vi "remote.Abort Session.vi"(8 "error in (no error)":errorcluster, 11 "SLSC Remote in":refnum<class "SLSC Interface.lvclass">) -> (0 "error out":errorcluster, 3 "SLSC Remote out":refnum<class "SLSC Interface.lvclass">)   [LabVIEW 2016, in "SLSC Interface.lvclass"]
uses:
  SLSC Interface Class/SLSC Interface.lvclass
  SLSC Interface Class/SLSC Interface.lvclass/SLSC Interface.ctl
  SLSC Interface Class/Read client handle.vi
  SLSC Interface Class/Read URL.vi
  <vilib>/NI/JSON Support for LabVIEW/JSON Data Classes/JSON Object/JSON Object.lvclass
  C:/Program Files (x86)/National Instruments/LabVIEW 2016/vi.lib/NI/JSON Support for LabVIEW/JSON Data Classes/JSON Datatype/JSON Null.lvclass
  SLSC Interface Class/Read session.vi
  <vilib>/NI/JSON Support for LabVIEW/JSON Data Classes/JSON Object/New JSON Object (Empty).vi
  <vilib>/NI/JSON Support for LabVIEW/JSON Data Classes/JSON Object/Insert Key Value Pair (Single String).vi
  <vilib>/NI/NI JSONRPC Server Framework/Classes/Server/Format Client Request (Auto-Increment).vi
  <vilib>/httpClient/POSTBuffer.vi
  <vilib>/NI/NI JSONRPC Server Framework/Classes/Server/Parse Response (Object).vi
  <vilib>/NI/NI JSONRPC Server Framework/Classes/Server/JSONRPC Server.lvclass
  <vilib>/httpClient/LabVIEWHTTPClient.lvlib
  <vilib>/NI/JSON Support for LabVIEW/JSON Data Classes/JSON Helper/JSON Helper.lvclass
  C:/Program Files (x86)/National Instruments/LabVIEW 2016/vi.lib/NI/JSON Support for LabVIEW/JSON Data Classes/JSON Structured Type/JSON Structure.lvclass
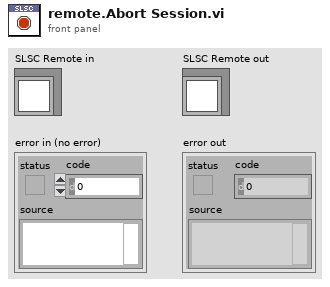
[diagram p1: front panel]
types:
  T1 = typedef "LabVIEWHTTPClient.lvlib/ClientHandle.ctl" = refnum<k1>
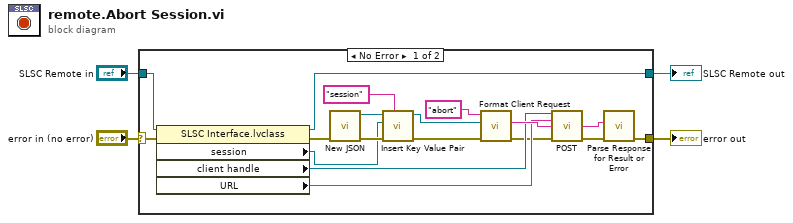
[diagram p0: block diagram]
diagram:
  n1 = case shown="No Error" "error in (no error)" {
    selector: "error in (no error)" -> [w20 w23]
    tunnel: "SLSC Remote in" -> [w22 w24]
    tunnel: [w21 w24] -> w2
    tunnel: [w8 w23] -> w1
    frame No Error {
      n2 = property class="SLSC Interface.lvclass"(reference=w22, error in=w20) -> (reference out=w21:refnum<class "SLSC Interface.lvclass">, error out=w19:errorcluster, "session"=w7:refnum<k21>, "client handle"=w13:T1, "URL"=w12:string)
      n3 = call-poly <vilib>:"New JSON.vi"("error in (no error)"=w19) -> ("error out"=w18:errorcluster, "JSON Object out"=w5:refnum<class "JSON Object.lvclass">)  [unwired: 9 in]
      n4 = call-poly <vilib>:"Insert Key Value Pair.vi"("key"="session" ("Name"), "error in (no error)"=w18, "value"=w7, "JSON Object in"=w5) -> ("error out"=w14:errorcluster, "JSON Object out"=w15:refnum<class "JSON Object.lvclass">)  [unwired: 5 in, 1 out]
      n5 = call-poly <vilib>:"Format Client Request.vi"("error in (no error)"=w14, "JSON in"=w15, "method"="abort") -> ("error out"=w11:errorcluster, "Request String"=w16:string)  [unwired: 7 in]
      n6 = call-poly <vilib>:"POST.vi"("client handle"=w13, "url"=w12, "buffer"=w16, "error in (no error)"=w11) -> ("body"=w10:string, "error out"=w9:errorcluster)  [unwired: 8 in, 2 out]
      n7 = call-poly <vilib>:"Parse Response for Result or Error.vi"("error in"=w9, "Response String In"=w10) -> ("error out"=w8:errorcluster)  [unwired: 7 in, 2 out]
    }
    frame Error {
    }
  }
  "error out" <- w1
  "SLSC Remote out" <- w2
